vi "TDT-Wait Sys Mode.vi"(0 "Data":T2={"TTankX"=refnum, "TDevAccX"=refnum, "LastTime"=0.0, "error"={"status"=FALSE, "code"=0, "source"=""}, "Block Name"="", "Circuit Tag"="", "Tank Name"="", "NumTicks"=0, "LastTick"=0.0, "Idle?"=FALSE, "Wait (ms)"=1000, "LastArtf"=0.0, "LastTosc"=0.0}, 7 "NewMode":T1, 11 "error in (no error)":errorcluster, 12 "milliseconds to wait":u32=1000) -> (15 "error out":errorcluster)   [LabVIEW 2015]
uses:
  TDT Interface Data.ctl
  TDT-Sys Mode Enum.ctl
panel:
  in  "Poll Interval (s)":dbl=0.1
  in  "Timeout (s)":dbl=2.0
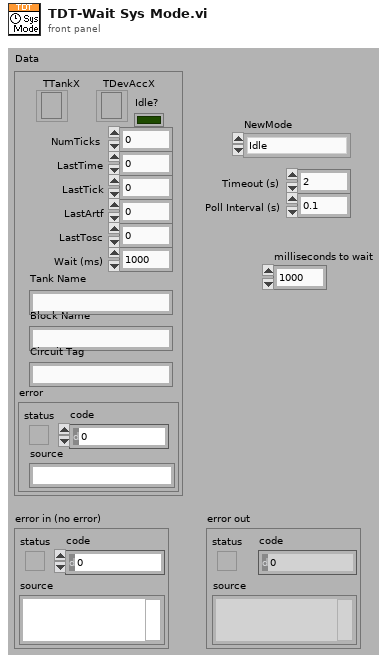
[diagram p1: front panel]
types:
  T1 = typedef "TDT-Sys Mode Enum.ctl" = enum16{"Idle", "Standby", "Preview", "Record"}
  T2 = typedef "TDT Interface Data.ctl" = cluster{"TTankX":refnum<k7>, "TDevAccX":refnum<k7>, "LastTime":dbl, "error":errorcluster, "Block Name":string, "Circuit Tag":string, "Tank Name":string, "NumTicks":i32, "LastTick":dbl, "Idle?":bool, "Wait (ms)":u32, "LastArtf":dbl, "LastTosc":dbl}
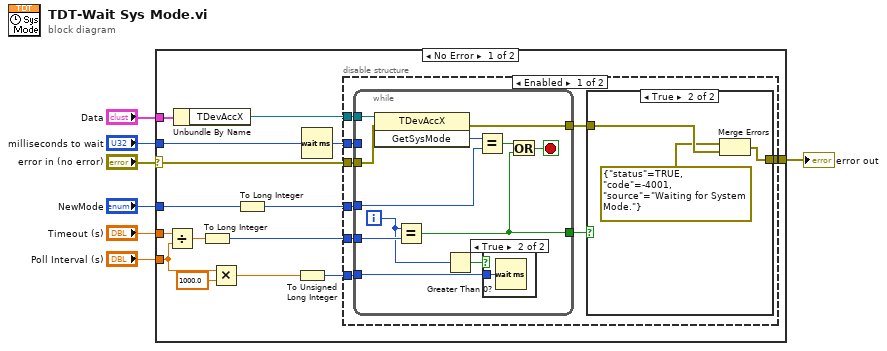
[diagram p0: block diagram]
diagram:
  n1 = case shown="No Error" "error in (no error)" {
    selector: "error in (no error)" -> [w10 w50]
    tunnel: [w11 w50] -> w6
    tunnel: "Data" -> [w22 _]
    tunnel: "NewMode" -> [w21 _]
    tunnel: "Timeout (s)" -> [w17 _]
    tunnel: "Poll Interval (s)" -> [w16 _]
    tunnel: "milliseconds to wait" -> [w9 _]
    frame No Error {
      n2 = Divide(x=w17, y=w16) -> (x/y=w18:dbl)
      n3 = Unbundle By Name(w22) -> ("TDevAccX"=w15:refnum<k7>)
      n4 = To Long Integer(number=w18) -> (32bit integer=w13:i32)
      n5 = Multiply(x=w16, y=1000.0) -> (x*y=w19:dbl)
      n6 = To Long Integer(number=w21) -> (32bit integer=w14:i32)
      n7 = To Unsigned Long Integer(number=w19) -> (unsigned 32bit integer=w12:u32)
      n8 = Wait (ms)(milliseconds to wait=w9) -> (millisecond timer value=w8:u32)
      n9 = disable-structure shown="Enabled" {
        disable-tunnel: w15 -> [w31 _]
        disable-tunnel: w14 -> [w30 _]
        disable-tunnel: w13 -> [w29 _]
        disable-tunnel: w12 -> [w28 _]
        disable-tunnel: [w26 w49] -> w11
        disable-tunnel: w10 -> [w24 w49]
        disable-tunnel: w8 -> [w23 _]
        frame Enabled {
          n10 = while {
            tunnel: w31 -> [w47]
            tunnel: w28 -> [w46]
            tunnel: w30 -> [w44]
            tunnel: w29 -> [w43]
            tunnel: w24 -> [w40]
            tunnel: [w39] -> w25
            tunnel: [w38] -> w27
            tunnel: w23 -> [_]
            i -> [w36]
            stop <- w41 stop-if-true
            n11 = invoke class="TDevAccX" method="GetSysMode"(reference=w47, error in=w40) -> (error out=w39:errorcluster, "GetSysMode"=w45:i32)  [unwired: 1 in, 1 out]
            n12 = Equal?(x=w36, y=w43) -> (x = y?=w38:bool)
            n13 = Greater Than 0?(x=w36) -> (x > 0?=w37:bool)
            n14 = Equal?(x=w45, y=w44) -> (x = y?=w42:bool)
            n15 = case shown="True" w37 {
              tunnel: w46 -> [_ w48]
              frame False {
              }
              frame True {
                n16 = Wait (ms)(milliseconds to wait=w48) -> ()  [unwired: 1 out]
              }
            }
            n17 = Or(x=w42, y=w38) -> (x .or. y?=w41:bool)
          }
          n18 = case shown="True" w27 {
            tunnel: [w32 w35] -> w26
            tunnel: w25 -> [w32 w34]
            frame False {
            }
            frame True {
              n19 = Merge Errors(errorcluster {"status"=TRUE, "code"=-4001, "source"="Waiting for System Mode."} ("error in 1 (no error)"), w34) -> (w35:errorcluster)
            }
          }
        }
        frame Disabled {
        }
      }
    }
    frame Error {
    }
  }
  "error out" <- w6
